vi "UpdateProgressBar.vi"(2 "error in":errorcluster, 3 "PBarValue":i32, 4 "reference in":refnum<vi>) -> (0 "error out":errorcluster, 1 "reference out":refnum<vi>)   [LabVIEW 2020]
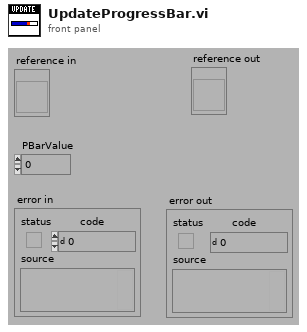
[diagram p1: front panel]
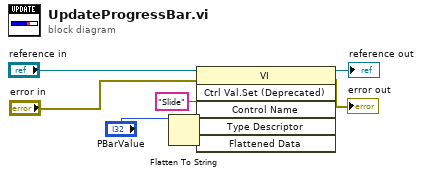
[diagram p0: block diagram]
diagram:
  n1 = Flatten To String(anything="PBarValue") -> (data string=w4:string, type string=w3:i16[])  [unwired: 3 in, 1 out]
  n2 = invoke class="VI" method="Ctrl Val.Set (Deprecated)"(reference="reference in", error in="error in", "Control Name"="Slide", "Type Descriptor"=w3, "Flattened Data"=w4) -> (reference out=→"reference out":refnum<vi>, error out=→"error out":errorcluster)  [unwired: 1 in, 4 out]
